vi "Calculate Offset Position.vi"(5 "Arc Length (degrees)":dbl format="%#_13g", 7 "Start Angle (degrees)":dbl format="%#_13g", 10 "Offset":i16=10, 11 "Original Position":cluster{"horizontal":i16, "vertical":i16}) -> (3 "Offset Position":cluster{"horizontal":i16, "vertical":i16})   [LabVIEW 2020, in "PieChart.lvclass"]
uses:
  PieChart.lvclass
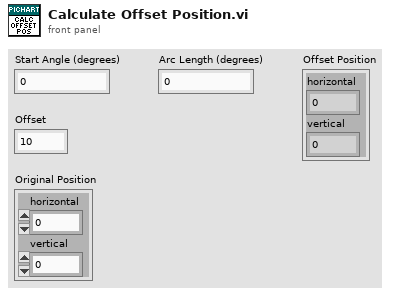
[diagram p1: front panel]
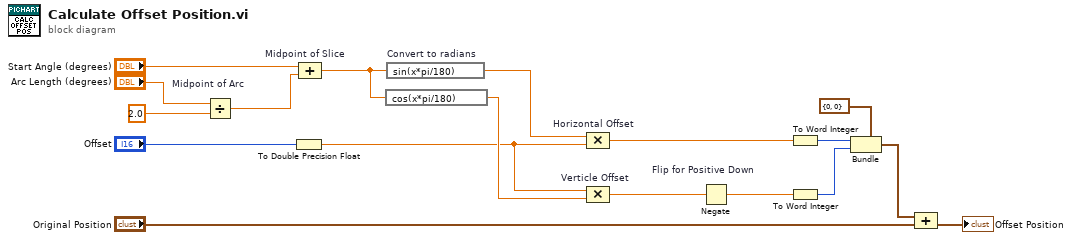
[diagram p0: block diagram]
diagram:
  n1 = Divide "Midpoint of Arc"(x="Arc Length (degrees)", y=2.0) -> (x/y=w5:dbl)
  n2 = To Double Precision Float(number="Offset") -> (double precision float=w1:dbl)
  n3 = Compound Arithmetic op=ADD "Midpoint of Slice"("Start Angle (degrees)", w5) -> (w4:dbl)
  n4 = expression code="cos(x*pi/180)"(w4) -> (w15:dbl)
  n5 = expression code="sin(x*pi/180)" "Convert to radians"(w4) -> (w17:dbl)
  n6 = Compound Arithmetic op=MULTIPLY "Horizontal Offset"(w17, w1) -> (w10:dbl)
  n7 = Compound Arithmetic op=MULTIPLY "Verticle Offset"(w1, w15) -> (w11:dbl)
  n8 = Negate "Flip for Positive Down"(x=w11) -> (-x=w9:dbl)
  n9 = To Word Integer(number=w10) -> (16bit integer=w3:i16)
  n10 = To Word Integer(number=w9) -> (16bit integer=w2:i16)
  n11 = Bundle(cluster=cluster{"horizontal":i16, "vertical":i16} {"horizontal"=0, "vertical"=0} ("pixel center"), "horizontal"=w3, "vertical"=w2) -> (w13:cluster{"horizontal":i16, "vertical":i16})
  n12 = Compound Arithmetic op=ADD(w13, "Original Position") -> (→"Offset Position":cluster{"horizontal":i16, "vertical":i16})
